vi "Query Conditions.vi"() -> ()   [LabVIEW 2024]
uses:
  <vilib>/Plug-In SDKs/Clients/Data Store V1/Data Store Client.lvlibp/API/Data Store V1/Read Data from Condition (Double Array).vi
  <vilib>/Plug-In SDKs/Clients/Data Store V1/Data Store Client.lvlibp
panel:
  in  "odata query":string="$filter=contains(Name,'Temperature') or contains(Name,'Pressure')"
  out "Filtered conditions":T1(array[cluster])
  out "error out":errorcluster
  # "Query Conditions\n\nThis example shows you to use odata to query for published conditions.\nRun Publish Data.vi to create the data that is queried by this VI."
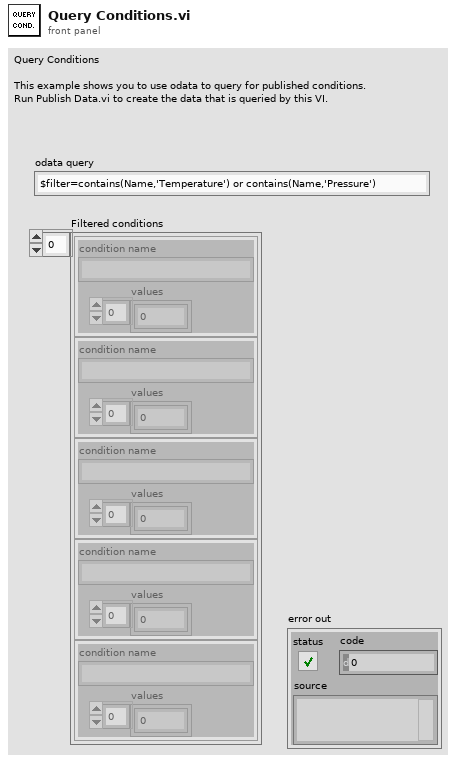
[diagram p1: front panel]
types:
  T1 = cluster{"condition name":string, "values":dbl[]}[]
  T2 = typedef "Data Store Client.lvlibp/Published Condition.ctl" = cluster{"moniker":T3, "published condition id":string, "condition name":string, "condition type":string, "step id":string, "test result id":string}
  T3 = typedef "Data Store Client.lvlibp/Data Moniker.ctl" = cluster{"service location":string, "data source":string, "data instance":i64}
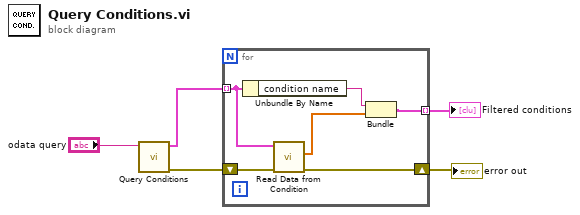
[diagram p0: block diagram]
diagram:
  n1 = call <vilib>:"Query Conditions.vi"("odata query"="odata query") -> ("error out"=w4:errorcluster, "stored condition values"=w1:T2[])  [unwired: 9 in]
  n2 = for {
    tunnel: w1 -> [w6] mode=indexing
    shift-right: [w10] -> w2
    shift-left: w4 -> [w11]
    tunnel: [w7] -> w3 mode=indexing
    n3 = Unbundle By Name(w6) -> ("condition name"=w9:string)
    n4 = call-poly <vilib>:"Read Data from Condition.vi"("error in"=w11, "published condition"=w6) -> ("error out"=w10:errorcluster, "values"=w8:dbl[])  [unwired: 6 in, 2 out]
    n5 = Bundle("condition name"=w9, "values"=w8) -> (w7:cluster{"condition name":string, "values":dbl[]})  [unwired: 1 in]
  }
  "error out" <- w2
  "Filtered conditions" <- w3
